vi "Write SP_Set.vi"(8 "error in (no error)":errorcluster, 9 "SP":dbl, 10 "SP_Set":dbl, 11 "Y_H in":refnum<class "Y_H.lvclass">) -> (0 "error out":errorcluster, 3 "Y_H out":refnum<class "Y_H.lvclass">)   [LabVIEW 2019, in "Y_H.lvclass"]
uses:
  Y_H.lvclass
  Y_H.lvclass/Y_H.ctl
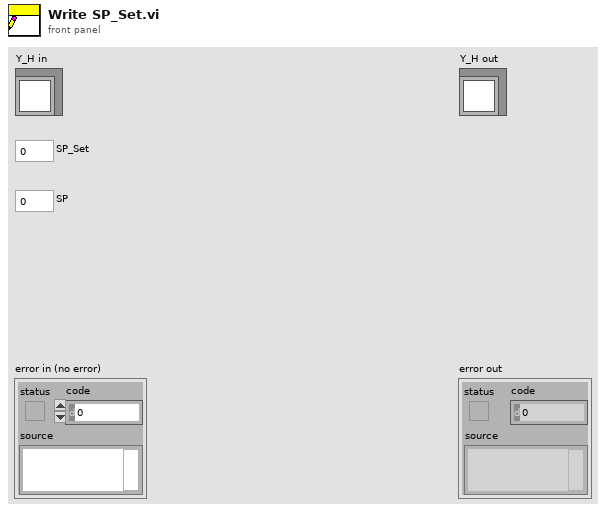
[diagram p1: front panel]
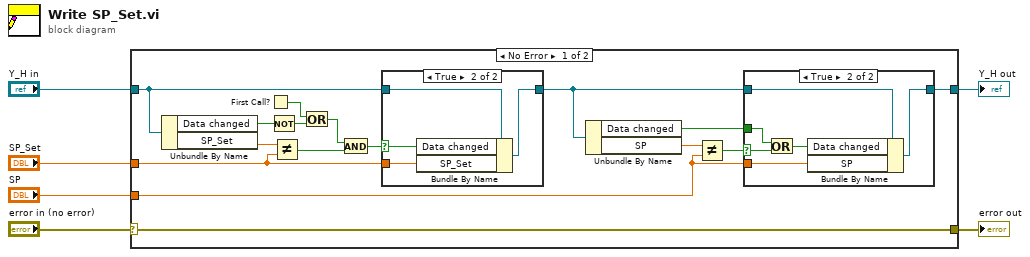
[diagram p0: block diagram]
diagram:
  n1 = case shown="No Error" "error in (no error)" {
    selector: "error in (no error)" -> [w22 w35]
    tunnel: [w22 w35] -> w5
    tunnel: [w9 w36] -> w3
    tunnel: "Y_H in" -> [w21 w36]
    tunnel: "SP_Set" -> [w19 _]
    tunnel: "SP" -> [w12 _]
    frame No Error {
      n2 = Unbundle By Name(w21) -> ("Data changed"=w16:bool, "SP_Set"=w20:dbl)
      n3 = First Call?() -> (First Call?: T/F=w8:bool)
      n4 = Not(x=w16) -> (.not. x?=w10:bool)
      n5 = Not Equal?(x=w20, y=w19) -> (x != y?=w18:bool)
      n6 = Or(x=w8, y=w10) -> (x .or. y?=w7:bool)
      n7 = And(x=w7, y=w18) -> (x .and. y?=w17:bool)
      n8 = case shown="True" w17 {
        selector: w17 -> [_ w31]
        tunnel: [w30 w34] -> w13
        tunnel: w21 -> [w30 w33]
        tunnel: w19 -> [_ w32]
        frame False {
        }
        frame True {
          n9 = Bundle By Name(cluster=w33, "Data changed"=w31, "SP_Set"=w32) -> (w34:refnum<class "Y_H.lvclass">)
        }
      }
      n10 = Unbundle By Name(w13) -> ("Data changed"=w11:bool, "SP"=w15:dbl)
      n11 = Not Equal?(x=w15, y=w12) -> (x != y?=w14:bool)
      n12 = case shown="True" w14 {
        selector: w14 -> [_ w26]
        tunnel: [w23 w29] -> w9
        tunnel: w13 -> [w23 w28]
        tunnel: w12 -> [_ w27]
        tunnel: w11 -> [_ w24]
        frame False {
        }
        frame True {
          n13 = Or(x=w24, y=w26) -> (x .or. y?=w25:bool)
          n14 = Bundle By Name(cluster=w28, "Data changed"=w25, "SP"=w27) -> (w29:refnum<class "Y_H.lvclass">)
        }
      }
    }
    frame Error {
    }
  }
  "error out" <- w5
  "Y_H out" <- w3
